vi "Get Cluster Element Names.vi"(11 "Cluster":variant) -> (3 "Channels":string[](array[string]))   [LabVIEW 2020, in "FPGA Addon System Explorer.lvlib"]
uses:
  FPGA Addon System Explorer.lvlib
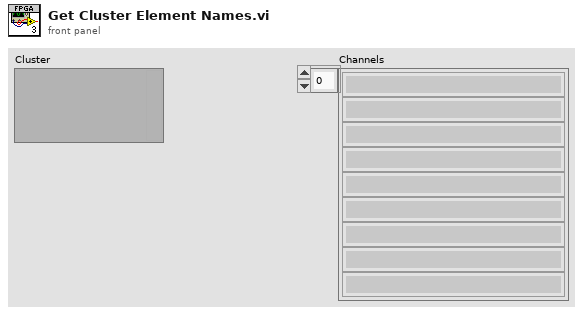
[diagram p1: front panel]
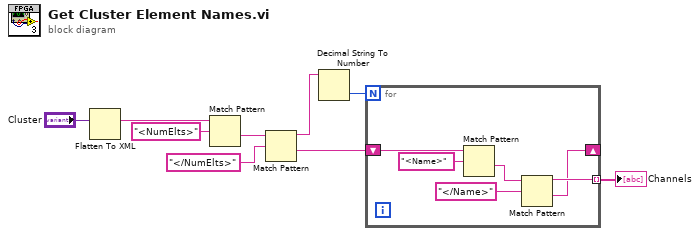
[diagram p0: block diagram]
diagram:
  n1 = Flatten To XML(6:"Cluster") -> (2:w8:string)
  n2 = Match Pattern(string=w8, regular expression="<NumElts>") -> (after substring=w9:string)  [unwired: 1 in, 3 out]
  n3 = Match Pattern(string=w9, regular expression="</NumElts>") -> (before substring=w5:string, after substring=w4:string)  [unwired: 1 in, 2 out]
  n4 = Decimal String To Number(string=w5) -> (number=w2:i32)  [unwired: 2 in, 1 out]
  n5 = for {
    N: w2 -> [_]
    tunnel: [w11] -> w3 mode=indexing
    shift-right: [w10] -> _
    shift-left: w4 -> [w12]
    n6 = Match Pattern(string=w12, regular expression="<Name>") -> (after substring=w15:string)  [unwired: 1 in, 3 out]
    n7 = Match Pattern(string=w15, regular expression="</Name>") -> (before substring=w11:string, after substring=w10:string)  [unwired: 1 in, 2 out]
  }
  "Channels" <- w3
